vi "batch_code.vi"(10 "shift":string) -> (2 "batch code o/P":string)   [LabVIEW 2017]
panel:
  out "date time rec":T1
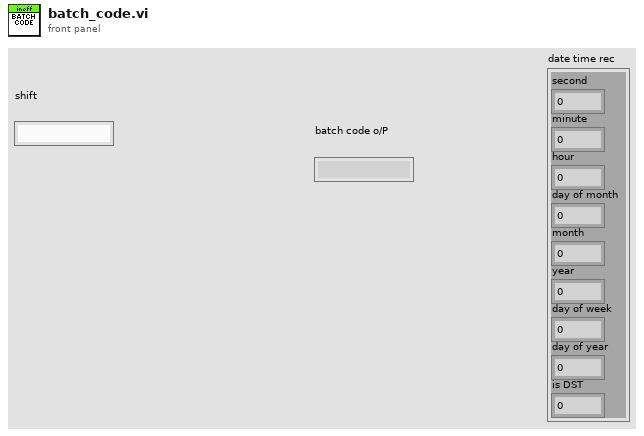
[diagram p1: front panel]
types:
  T1 = cluster{"second":i32, "minute":i32, "hour":i32, "day of month":i32, "month":i32, "year":i32, "day of week":i32, "day of year":i32, "is DST":i32}
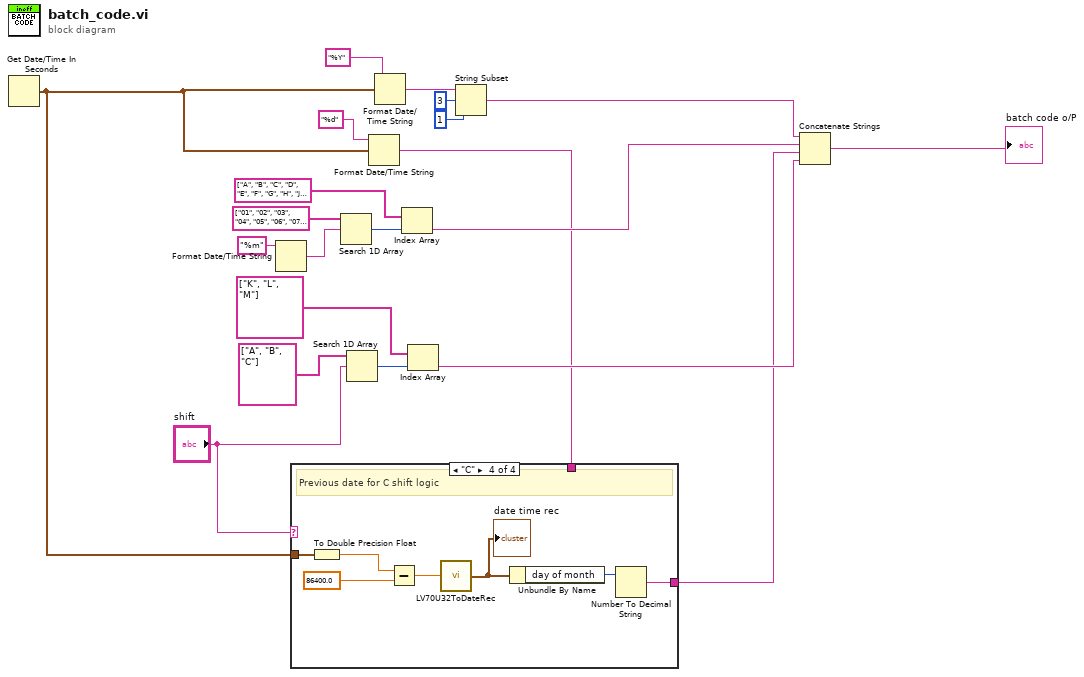
[diagram p0: block diagram]
diagram:
  n1 = Get Date/Time In Seconds() -> (seconds since 1Jan1904=w4:timestamp)
  n2 = Format Date/Time String(time format string (%c)="%m") -> (date/time string=w14:string)  [unwired: 2 in]
  n3 = Search 1D Array(1D array=string[] ["01", "02", "03", "04", "05", "06", "07", "08", "09", "10", "11", "12"], element=w14) -> (index of element=w13:i32)  [unwired: 1 in]
  n4 = Search 1D Array(1D array=string[] ["A", "B", "C"], element="shift") -> (index of element=w8:i32)  [unwired: 1 in]
  n5 = Format Date/Time String(time format string (%c)="%d", seconds (now)=w4) -> (date/time string=w1:string)  [unwired: 1 in]
  n6 = case shown="\"C\"" "shift" {
    tunnel: w4 -> [_ _ _ w28]
    tunnel: [w22 w23 w24 w25] -> w2
    tunnel: w1 -> [w22 w23 w24 _]
    frame "False", Default {
    }
    frame "A" {
    }
    frame "B" {
    }
    frame "C" {
      # "Previous date for C shift logic"
      n7 = To Double Precision Float(number=w28) -> (double precision float=w29:dbl)
      n8 = Subtract(x=w29, y=86400.0) -> (x-y=w30:dbl)
      n9 = call <vilib>:"LV70U32ToDateRec.vi"("Time"=w30) -> ("date time rec"=w31:T1)
      "date time rec" <- w31
      n10 = Unbundle By Name(w31) -> ("day of month"=w26:i32)
      n11 = Number To Decimal String(number=w26) -> (decimal integer string=w25:string)  [unwired: 1 in]
    }
  }
  n12 = Format Date/Time String(time format string (%c)="%Y", seconds (now)=w4) -> (date/time string=w20:string)  [unwired: 1 in]
  n13 = Index Array(array=string[] ["A", "B", "C", "D", "E", "F", "G", "H", "J", "K", "L", "M"], index=w13) -> (element=w5:string)
  n14 = Index Array(array=string[] ["K", "L", "M"], index=w8) -> (element=w6:string)
  n15 = String Subset(string=w20, offset (0)=3, length (rest)=1 ("length (rest)")) -> (substring=w11:string)
  n16 = Concatenate Strings(w11, w5, w2, w6) -> (→"batch code o/P":string)
